vi "CANOpen_Main_Set Node State.vi"(6 "Start NMT":bool, 8 "error in (no error)":errorcluster, 10 "Nodes":T2[](array[typedef]) {"NMT"."Node init static SDO state" items=["start remote node"=1, "enter pre-operational"=128]; "NMT"."Node run state" items=["start remote node"=1, "stop remote node"=2, "enter pre-operational"=128, "reset node"=129, "reset communication"=130]; "Dynamic SDOs"."Sub-Index (0)" format="%.0x"; "Dynamic SDOs"."Object Index" format="%.0x"; "Dynamic SDOs"."Block Data" format="%.0x"; "RPDOs"."PDO Channel" items=["PDO 1", "PDO 2", "PDO 3", "PDO 4"]; "RPDOs"."Parameters"."Bit Offset" max=8 step=1; "RPDOs"."Parameters"."Byte Offset" max=8 step=1; "TPDOs"."PDO Channel" items=["PDO 1", "PDO 2", "PDO 3", "PDO 4"]; "TPDOs"."Parameters"."Bit Offset" max=8 step=1; "TPDOs"."Parameters"."Byte Offset" max=8 step=1; "SDOs"."Sub-Index (0)" format="%.0x"; "SDOs"."Object Index" format="%.0x"; "SDOs"."Block Data" format="%.0x"}, 11 "interface object":refnum<k20>) -> (0 "error out":errorcluster, 1 "States":u16[](array[ring]) items=["unknown"=1, "bootup"=0, "stopped"=4, "operational"=5, "pre-operational"=127, "connection lost"=128], 3 "interface object out":refnum<k20>, 5 "Security Ref":T1)   [LabVIEW 2013, in "CANOpen Addon Custom Device.lvlib"]
uses:
  CANOpen Addon Custom Device.lvlib
  SubVIS/CANOpen_Node Message Settings.ctl
  Shared Code/CANOpen_PDO Settings.ctl
  Shared Code/CANOpen_PDO Parameter Settings.ctl
  Shared Code/CANOpen_PDO Data Type.ctl
  System Explorer/SubVIs/CANopen Byte Order.ctl
  Shared Code/CANOpen_SDO Settings.ctl
  SubVIS/CANOpen_NMT Settings.ctl
  CanOpen_NMT_Config.ctl
  CanOpen_NMT_Static detect.ctl
  CANOpen_HB_NG_EM Refs.ctl
panel:
  # "LSB"
  # "MSB"
  # "LSB"
  # "MSB"
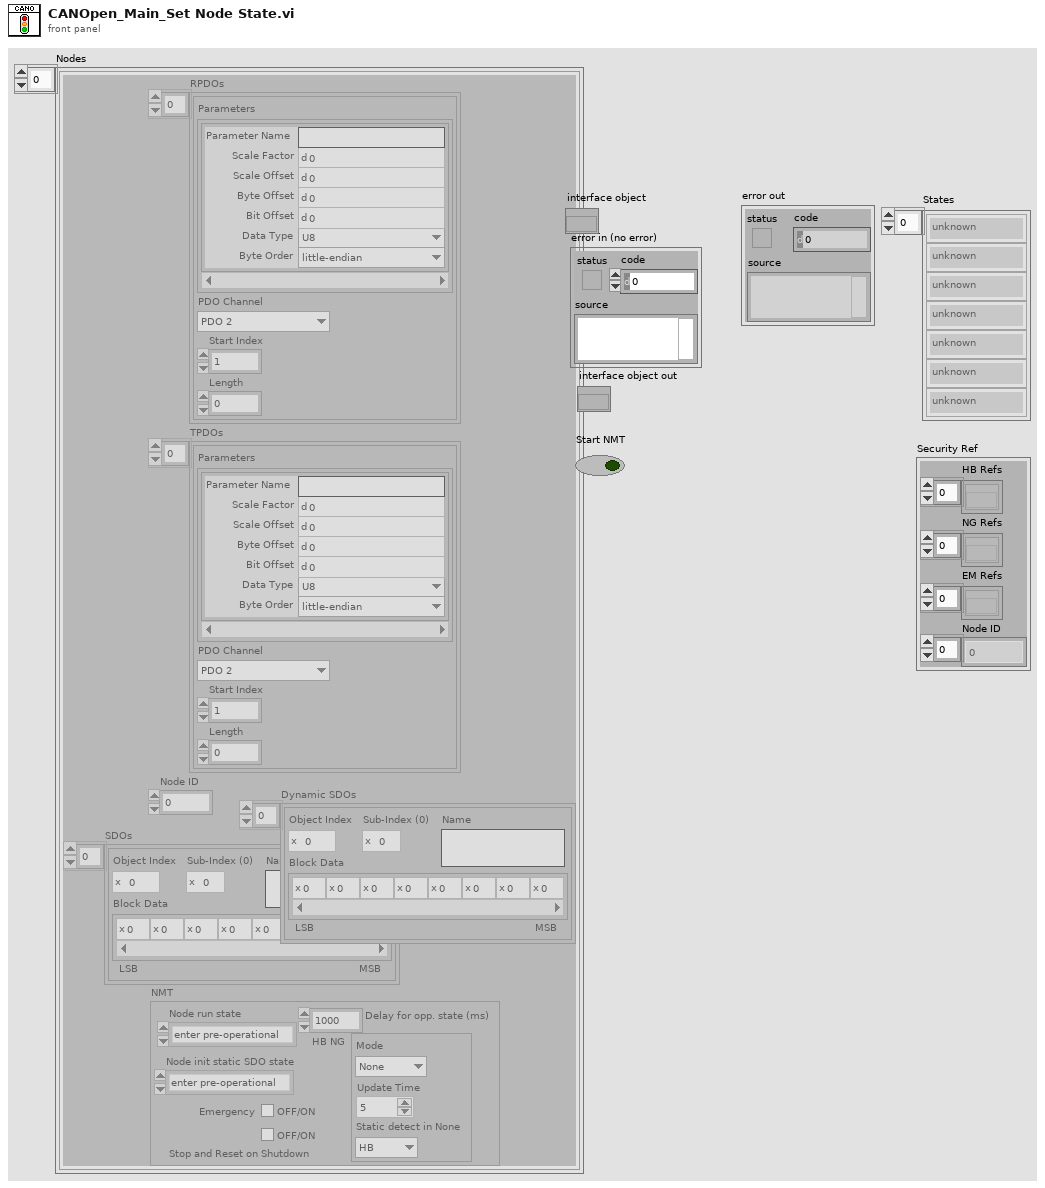
[diagram p1: front panel]
types:
  T1 = typedef "CANOpen Addon Custom Device.lvlib/CANOpen_HB_NG_EM Refs.ctl" = cluster{"HB Refs":refnum<k20>[], "NG Refs":refnum<k20>[], "EM Refs":refnum<k20>[], "Node ID":u8[]}
  T2 = typedef "CANOpen_Node Message Settings.ctl" = cluster{"RPDOs":T3[], "TPDOs":T3[], "Node ID":u8, "SDOs":T7[], "Dynamic SDOs":T7[], "NMT":T8}
  T3 = typedef "CANOpen Addon Custom Device.lvlib/CANOpen_PDO Settings.ctl" = cluster{"Parameters":T4[], "PDO Channel":u8, "Start Index":u32, "Length":u32}
  T4 = typedef "CANOpen Addon Custom Device.lvlib/CANOpen_PDO Parameter Settings.ctl" = cluster{"Parameter Name":string, "Scale Factor":dbl, "Scale Offset":dbl, "Byte Offset":u8, "Bit Offset":u8, "Data Type":T5, "Byte Order":T6}
  T5 = typedef "CANOpen Addon Custom Device.lvlib/CANOpen_PDO Data Type.ctl" = enum16{"U8", "U16", "U32", "I8", "I16", "I32", "Single", "Double", "Boolean"}
  T6 = typedef "CANOpen Addon Custom Device.lvlib/CANopen Byte Order.ctl" = enum16{"big-endian network order", "little-endian"}
  T7 = typedef "CANOpen Addon Custom Device.lvlib/CANOpen_SDO Settings.ctl" = cluster{"Object Index":u16, "Sub-Index (0)":u8, "Block Data":u8[], "Name":string}
  T8 = typedef "CANOpen Addon Custom Device.lvlib/CANOpen_NMT Settings.ctl" = cluster{"Node run state":u16, "Emergency":bool, "HB NG":T9, "Delay for opp. state (ms)":dbl, "Node init static SDO state":u16, "Stop and Reset on Shutdown":bool}
  T9 = typedef "CANOpen Addon Custom Device.lvlib/CanOpen_NMT_Config.ctl" = cluster{"Mode":T10, "Update Time":u16, "Static detect in None":T10}
  T10 = typedef "CANOpen Addon Custom Device.lvlib/CanOpen_NMT_Static detect.ctl" = enum16{"None", "HB", "NG"}
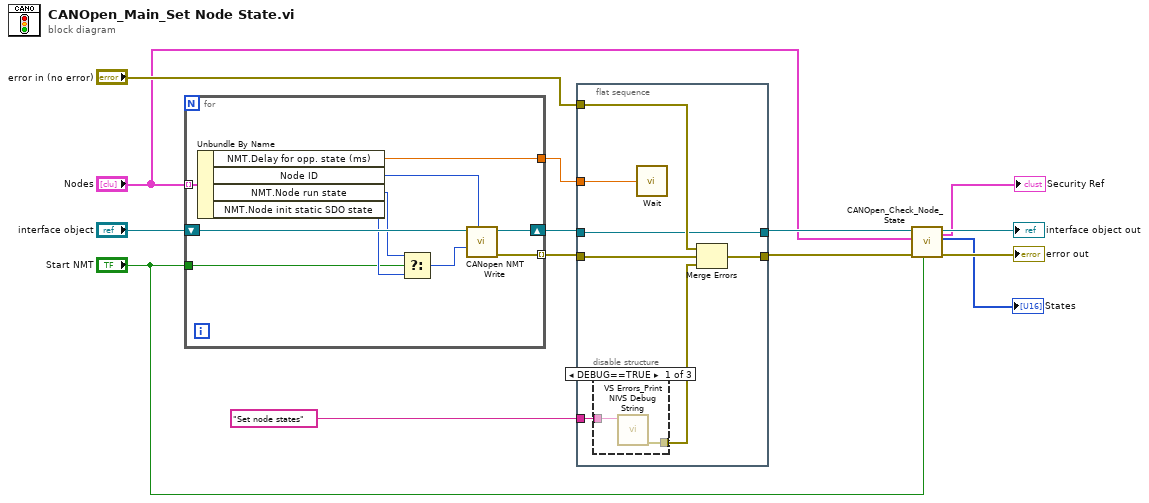
[diagram p0: block diagram]
diagram:
  n1 = for {
    shift-right: [w23] -> w10
    shift-left: "interface object" -> [w24]
    tunnel: "Nodes" -> [w22] mode=indexing
    tunnel: [w20] -> w12 mode=indexing
    tunnel: [w19] -> w3
    tunnel: "Start NMT" -> [w15]
    n2 = Unbundle By Name(w22) -> ("NMT.Delay for opp. state (ms)"=w19:dbl, "Node ID"=w21:u8, "NMT.Node run state"=w18:u16, "NMT.Node init static SDO state"=w17:u16)
    n3 = Select(t=w18, s=w15, f=w17) -> (s? t:f=w16:u16)
    n4 = call <vilib>:"CANopen NMT Write.vi"("node-ID (0)"=w21, "command"=w16, "interface object in"=w24) -> ("error out"=w20:errorcluster, "interface object out"=w23:refnum<k20>)  [unwired: 7 in]
  }
  n5 = flat-sequence {
    tunnel: [w28] -> w9
    tunnel: "Set node states" -> [w31]
    tunnel: w12 -> [w30]
    tunnel: "error in (no error)" -> [w27]
    tunnel: [w26] -> w7
    tunnel: w10 -> [w26]
    tunnel: w3 -> [w25]
    frame #0 {
      n6 = disable-structure shown="DEBUG==TRUE" {
        disable-tunnel: w31 -> [w33 _ _]
        disable-tunnel: [w32 _ _] -> w29
        frame condition #0 {
          n7 = call "VS Errors_Print NIVS Debug String.vi"("Debug String"=w33) -> ("error out"=w32:errorcluster)  [unwired: 9 in]
        }
        frame condition #1 {
        }
        frame condition #2 (active) {
        }
      }
      n8 = call "Wait"("Count(mSec)"=w25) -> ()  [unwired: 1 out]
      n9 = Merge Errors(w27, w30, w29) -> (w28:errorcluster)
    }
  }
  n10 = call "CANOpen_Check_Node_State.vi"("Start NMT"="Start NMT", "error in"=w9, "Nodes"="Nodes", "interface object"=w7) -> ("error out"=→"error out":errorcluster, "States"=→"States":u16[], "interface object out"=→"interface object out":refnum<k20>, "Security Ref"=→"Security Ref":T1)  [unwired: 4 in]
